vi "Create Analog DataSet MultiRow & ChanNames DataQ.vi"(8 "error in (no error)":errorcluster, 9 "Select":T1, 10 "TaskName":string, 11 "DataQueues in":refnum<class "DataQueues.lvclass">) -> (0 "error out":errorcluster, 2 "TaskName out":string, 3 "DataQueues out":refnum<class "DataQueues.lvclass">)   [LabVIEW 2017, in "DataQueues.lvclass"]
doc: "Developed by Kevin Thompson\nkevin@thompsonengineering.net\n\nCopyright 2018-2020\nThompson Engineering, LLC"
uses:
  DataQueues.lvclass
  DataTypes/DataQ SelectType--enum.ctl
  DataTypes/DataQ Ref DictNode--cluster.ctl
  DataTypes/Analog DataSet MultiRow & ChanNames--cluster.ctl
  DataQueues.lvclass/DataQueues.ctl
  Accessors/Get QueueNames.vi
  Accessors/Get DataQ Dict.vi
  Accessors/Set QueueNames.vi
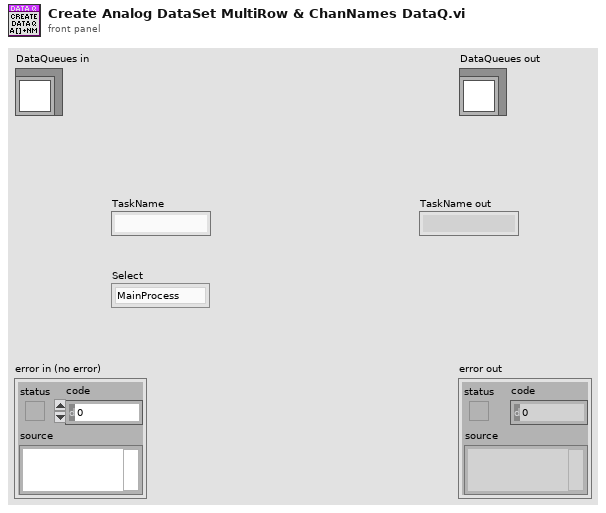
[diagram p1: front panel]
types:
  T1 = typedef "DataQueues.lvclass/DataQ SelectType--enum.ctl" = enum16{"MainProcess", "LogEngine", "LocalDAQThread"}
  T2 = typedef "DataQueues.lvclass/Analog DataSet MultiRow & ChanNames--cluster.ctl" = cluster{"TimeStamp_(s)":dbl, "data":dbl[][], "ChanNames":string[]}
  T3 = typedef "DataQueues.lvclass/DataQ Ref DictNode--cluster.ctl" = cluster{"KeyName":string, "Type Name":string, "vDataQ Ref":variant}
  T4 = typedef "TD Dynamic CVT DVR--ref.ctl" = refnum<data-value>
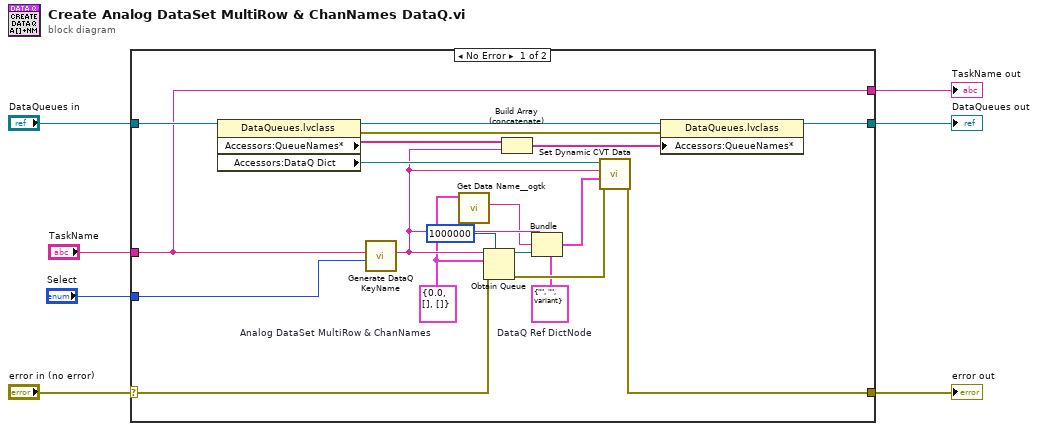
[diagram p0: block diagram]
diagram:
  n1 = case shown="No Error" "error in (no error)" {
    selector: "error in (no error)" -> [w24 w29]
    tunnel: [w23 w29] -> w6
    tunnel: [w22 w28] -> w4
    tunnel: "DataQueues in" -> [w20 w28]
    tunnel: "TaskName" -> [w9 w27]
    tunnel: "Select" -> [w26 _]
    tunnel: [w9 w27] -> w1
    frame No Error {
      w11 = T2 {"TimeStamp_(s)"=0.0, "data"=[], "ChanNames"=[]}  # Analog DataSet MultiRow & ChanNames
      w12 = T3 {"KeyName"="", "Type Name"="", "vDataQ Ref"=variant(refnum<queue> refnum)}  # DataQ Ref DictNode
      n2 = property class="DataQueues.lvclass"(reference=w20) -> (reference out=w19:refnum<class "DataQueues.lvclass">, error out=w10:errorcluster, "Accessors:QueueNames*"=w18:string[], "Accessors:DataQ Dict"=w21:T4)  [unwired: 1 in]
      n3 = call "Generate DataQ KeyName.vi"("Select"=w26, "TaskName"=w9) -> ("DataQ KeyName"=w15:string)  [unwired: 9 in]
      n4 = call <userlib>:"Get Data Name__ogtk.vi"("Data"=w11) -> ("Data Name"=w13:string)  [unwired: 8 in, 2 out]
      n5 = Obtain Queue(max queue size (-1, unlimited)=1000000, name (unnamed)=w15, element data type=w11, error in (no error)=w24) -> (queue out=w16:refnum<queue>, error out=w25:errorcluster)  [unwired: 1 in, 1 out]
      n6 = Build Array (concatenate)(w18, w15) -> (w17:string[])
      n7 = Bundle(cluster=w12, "KeyName"=w15, "Type Name"=w13, "vDataQ Ref"=w16) -> (w14:T3)
      n8 = call <vilib>:"Set Dynamic CVT Data.vi"("error in (no error)"=w25, "value"=w14, "DataName"=w15, "dCVT DVR"=w21) -> ("error out"=w23:errorcluster)  [unwired: 5 in, 2 out]
      n9 = property class="DataQueues.lvclass"(reference=w19, error in=w10, "Accessors:QueueNames*"=w17) -> (reference out=w22:refnum<class "DataQueues.lvclass">)  [unwired: 1 out]
    }
    frame Error {
    }
  }
  "error out" <- w6
  "DataQueues out" <- w4
  "TaskName out" <- w1
